vi "Test 3 Parse Response When Measuring Negative Voltage.vi"(8 "error in (no error)":errorcluster, 11 "Test Case In":refnum<class "Driver Test.lvclass">) -> (0 "error out":errorcluster, 3 "Test Case Out":refnum<class "Driver Test.lvclass">)   [LabVIEW 2020, in "Driver Test.lvclass"]
uses:
  Driver Test.lvclass
  Driver Test.lvclass/Driver Test.ctl
  Mock Serial.lvclass
  Driver/Driver.lvclass
  e83b171a-c1d6-4db8-9d64-19d6ae92fd3f.vi
  C:/git/astemes-lmock/sandbox/Examples/Serial/Serial.lvclass/Serial.lvclass
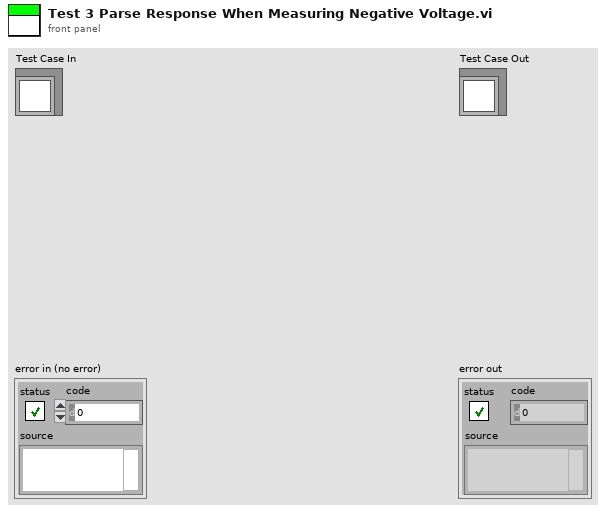
[diagram p1: front panel]
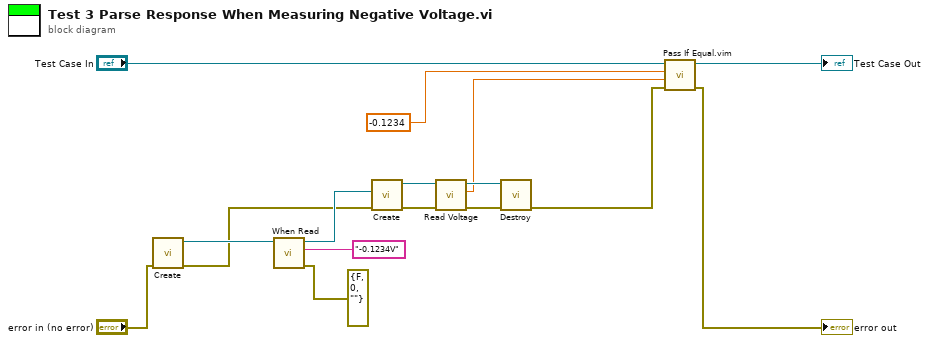
[diagram p0: block diagram]
diagram:
  n1 = call "Create.vi"("error in (no error)"="error in (no error)") -> ("error out"=w3:errorcluster, "Mock Class Generator out"=w5:refnum<class "Mock Serial.lvclass">)  [unwired: 9 in]
  n2 = call "When Read.vi"("error out"=errorcluster {"status"=FALSE, "code"=0, "source"=""}, "read buffer"="-0.1234V" ("write buffer"), "Serial in"=w5) -> ("Serial out"=w8:refnum<class "Mock Serial.lvclass">)  [unwired: 8 in]
  n3 = call "Create.vi"("error in (no error)"=w3, "Serial"=w8) -> ("error out"=w13:errorcluster, "Driver"=w11:refnum<class "Driver.lvclass">)  [unwired: 8 in]
  n4 = call "Read Voltage.vi"("error in (no error)"=w13, "Driver in"=w11) -> ("error out"=w12:errorcluster, "Voltage"=w1:dbl, "Driver out"=w10:refnum<class "Driver.lvclass">)  [unwired: 7 in]
  n5 = call "Destroy.vi"("error in (no error)"=w12, "Driver"=w10) -> ("error out"=w7:errorcluster)  [unwired: 9 in]
  n6 = call "Pass If Equal.vim"("error in (no error)"=w7, "Actual"=w1, "Expected"=-0.1234, "LUnit Test Case In"="Test Case In") -> ("error out"=→"error out":errorcluster, "LUnit Test Case Out"=→"Test Case Out":refnum<class "Driver Test.lvclass">)  [unwired: 6 in]
